vi "write_signal_hdf5.vi"(7 "Index":i32, 8 "error in":errorcluster, 9 "File Name":string="\\", 10 "Save Path":path, 11 "Signal array":T2[](array[typedef])) -> (0 "error out":errorcluster, 3 "Signal Processing:":T4={"Integer Timestamp"=0, "Dust Event ID"=0, "Role ID"=enum."First_Detector", "Data"=[], "Signal Length"=0, "dt"=0.0, "Offset"=0.0, "Hardware ID"=enum."CSA 1"})   [LabVIEW 2013]
uses:
  Public API/Post_Signal.ctl
  Role ID.ctl
  Hardware ID.ctl
  Public API/Signal.ctl
  <vilib>/addons/h5labview/polymorph/H5D_write_var.vi
  <vilib>/addons/h5labview/H5Dataset.lvlib
  <vilib>/addons/h5labview/H5Attrib.lvlib
panel:
  out "concatenated string":string
  out "Role ID":T1
  # "Signal"
  # "Signal"
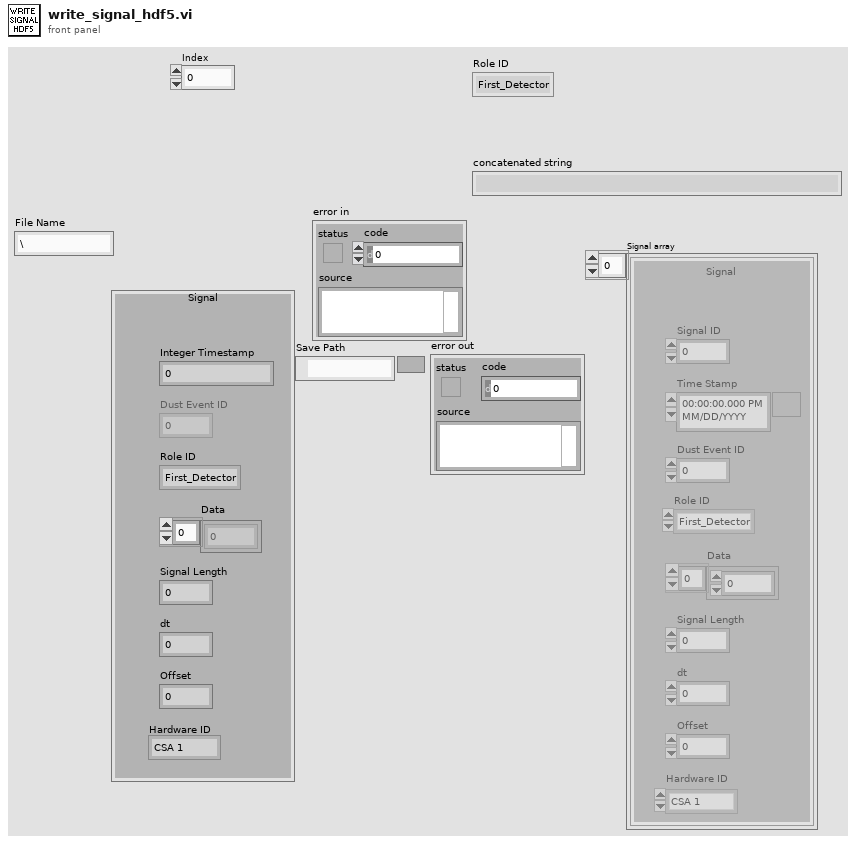
[diagram p1: front panel]
types:
  T1 = typedef "Role ID.ctl" = enum16{"First_Detector", "Second_Detector", "Third_Detector", "LeCroy_CH1", "LeCroy_CH2", "LeCroy_CH3", "LeCroy_CH4", "PSU"}
  T2 = typedef "Signal.ctl" = cluster{"Signal ID":i64, "Time Stamp":timestamp, "Dust Event ID":i64, "Role ID":T1, "Data":sgl[], "Signal Length":i32, "dt":sgl, "Offset":dbl, "Hardware ID":T3}
  T3 = typedef "Hardware ID.ctl" = enum16{"Unknown", "CSA 1", "CSA 2", "CSA 3", "CSA 4", "CSA 5", "CSA 6"}
  T4 = typedef "Post_Signal.ctl" = cluster{"Integer Timestamp":i64, "Dust Event ID":i64, "Role ID":T1, "Data":sgl[], "Signal Length":i32, "dt":sgl, "Offset":dbl, "Hardware ID":T3}
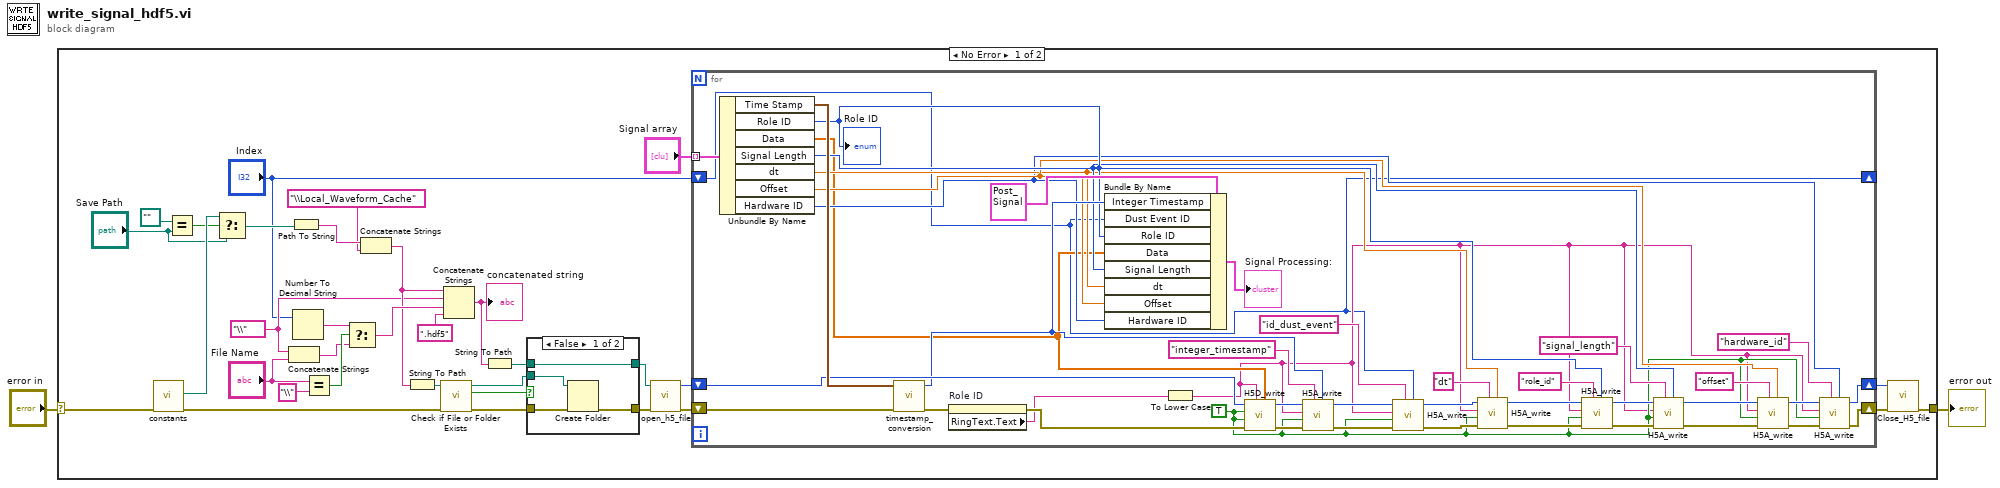
[diagram p0: block diagram]
diagram:
  n1 = case shown="No Error" "error in" {
    selector: "error in" -> [w27 w84]
    tunnel: [w29 w84] -> w1
    frame No Error {
      w5 = "\\"
      n2 = call "constants.vi"("error in (no error)"=w27) -> ("error out"=w11:errorcluster, "file path for Signal .hdf5 files"=w24:path)  [unwired: 4 in, 5 out]
      n3 = Equal?(x=path "" ("Save Path"), y="Save Path") -> (x = y?=w23:bool)
      n4 = Select(t=w24, s=w23, f="Save Path") -> (s? t:f=w26:path)
      n5 = Concatenate Strings(w5, "File Name") -> (w19:string)
      n6 = Path To String(path=w26) -> (string=w15:string)
      n7 = Number To Decimal String(number="Index") -> (decimal integer string=w17:string)  [unwired: 1 in]
      n8 = Equal?(x="File Name", y="\\") -> (x = y?=w20:bool)
      n9 = Select(t=w17, s=w20, f=w19) -> (s? t:f=w16:string)
      n10 = Concatenate Strings(w15, "\\Local_Waveform_Cache" ("string")) -> (w10:string)
      n11 = String To Path(string=w10) -> (path=w9:path)
      n12 = call <vilib>:"Check if File or Folder Exists.vi"("error in (no error)"=w11, "path"=w9) -> ("error out"=w12:errorcluster, "file or folder exists?"=w14:bool, "dup path"=w13:path)  [unwired: 7 in]
      n13 = Concatenate Strings(w10, w5, w16, ".hdf5") -> (w33:string)
      "concatenated string" <- w33
      n14 = String To Path(string=w33) -> (path=w7:path)
      n15 = case shown="False" w14 {
        tunnel: w13 -> [w39 _]
        tunnel: w12 -> [w38 w41]
        tunnel: [w37 w41] -> w8
        tunnel: w7 -> [w36 w40]
        tunnel: [w36 w40] -> w6
        frame False {
          n16 = Create Folder(path (use dialog)=w39, error in=w38) -> (error out=w37:errorcluster)  [unwired: 1 in, 2 out]
        }
        frame True {
        }
      }
      n17 = call "open_h5_file.vi"("error in (no error)"=w8, "path"=w6) -> ("error out"=w34:errorcluster, "ref"=w32:i32)  [unwired: 8 in]
      n18 = for {
        tunnel: "Signal array" -> [w81] mode=indexing
        shift-right: [w55] -> w30
        shift-left: w34 -> [w80]
        shift-right: [w42] -> _
        shift-left: "Index" -> [w42]
        shift-right: [w54] -> w31
        shift-left: w32 -> [w77]
        w47 = TRUE ("preserve attribs?")
        n19 = Unbundle By Name(w81) -> ("Time Stamp"=w82:timestamp, "Role ID"=w66:T1, "Data"=w45:sgl[], "Signal Length"=w65:i32, "dt"=w48:sgl, "Offset"=w64:dbl, "Hardware ID"=w46:T3)
        "Role ID" <- w66
        n20 = call "timestamp_conversion.vi"("error in (no error)"=w80, "Time Stamp"=w82) -> ("error out"=w78:errorcluster, "Integer Time"=w72:i64)  [unwired: 7 in]
        n21 = property on="Role ID" class="Enum (strict)"(error in=w78) -> (error out=w76:errorcluster, "RingText.Text"=w44:string)  [unwired: 1 in, 1 out]
        n22 = Bundle By Name(cluster=T4 {"Integer Timestamp"=0, "Dust Event ID"=0, "Role ID"=enum."First_Detector", "Data"=[], "Signal Length"=0, "dt"=0.0, "Offset"=0.0, "Hardware ID"=enum."CSA 1"} ("Post_Signal 2"), "Integer Timestamp"=w72, "Dust Event ID"=w42, "Role ID"=w66, "Data"=w45, "Signal Length"=w65, "dt"=w48, "Offset"=w64, "Hardware ID"=w46) -> (→"Signal Processing:":T4)
        n23 = To Lower Case(string=w44) -> (all lower case string=w43:string)
        n24 = call-poly <vilib>:"H5D_write.vi"("data"=w45, "name"=w43, "error in (no error)"=w76, "overwrite?"=w47, "preserve attribs?"=w47, "ref"=w77) -> ("error out"=w74:errorcluster, "ref out"=w75:i32)  [unwired: 2 in]
        n25 = call <vilib>:"H5A_write.vi"("value"=w72, "attrib_name"="integer_timestamp", "error in (no error)"=w74, "overwrite? (F)"=w47, "obj_name"=w43, "ref"=w75) -> ("error out"=w60:errorcluster, "ref out"=w59:i32)  [unwired: 2 in]
        n26 = call <vilib>:"H5A_write.vi"("value"=w42, "attrib_name"="id_dust_event", "error in (no error)"=w60, "overwrite? (F)"=w47, "obj_name"=w43, "ref"=w59) -> ("error out"=w53:errorcluster, "ref out"=w50:i32)  [unwired: 2 in]
        n27 = call <vilib>:"H5A_write.vi"("value"=w48, "attrib_name"="dt", "error in (no error)"=w53, "overwrite? (F)"=w47, "obj_name"=w43, "ref"=w50) -> ("error out"=w52:errorcluster, "ref out"=w49:i32)  [unwired: 2 in]
        n28 = call <vilib>:"H5A_write.vi"("value"=w66, "attrib_name"="role_id", "error in (no error)"=w52, "overwrite? (F)"=w47, "obj_name"=w43, "ref"=w49) -> ("error out"=w61:errorcluster, "ref out"=w56:i32)  [unwired: 2 in]
        n29 = call <vilib>:"H5A_write.vi"("value"=w65, "attrib_name"="signal_length", "error in (no error)"=w61, "overwrite? (F)"=w47, "obj_name"=w43, "ref"=w56) -> ("error out"=w62:errorcluster, "ref out"=w57:i32)  [unwired: 2 in]
        n30 = call <vilib>:"H5A_write.vi"("value"=w64, "attrib_name"="offset", "error in (no error)"=w62, "overwrite? (F)"=w47, "obj_name"=w43, "ref"=w57) -> ("error out"=w63:errorcluster, "ref out"=w58:i32)  [unwired: 2 in]
        n31 = call <vilib>:"H5A_write.vi"("value"=w46, "attrib_name"="hardware_id", "error in (no error)"=w63, "overwrite? (F)"=w47, "obj_name"=w43, "ref"=w58) -> ("error out"=w55:errorcluster, "ref out"=w54:i32)  [unwired: 2 in]
      }
      n32 = call "Close_H5_file.vi"("error in (no error)"=w30, "ref"=w31) -> ("error out"=w29:errorcluster)  [unwired: 9 in]
    }
    frame Error {
    }
  }
  "error out" <- w1
